vi "WaveformDataTypeTest.vi"() -> ()   [LabVIEW 2017]
uses:
  <userlib>/_OpenG.lib/lvdata/lvdata.llb/Waveform Subtype Enum__ogtk.ctl
panel:
  out "Waveform Subtype Enum":T1 format="%.0x"
  out "StreamTrace":waveform(dbl)(graph)={"t0"=timestamp(1099.9 s since 1904-01-01), "dt"=0.09999999999990905, "Y"=array[30001 elements]} caption="Stream"
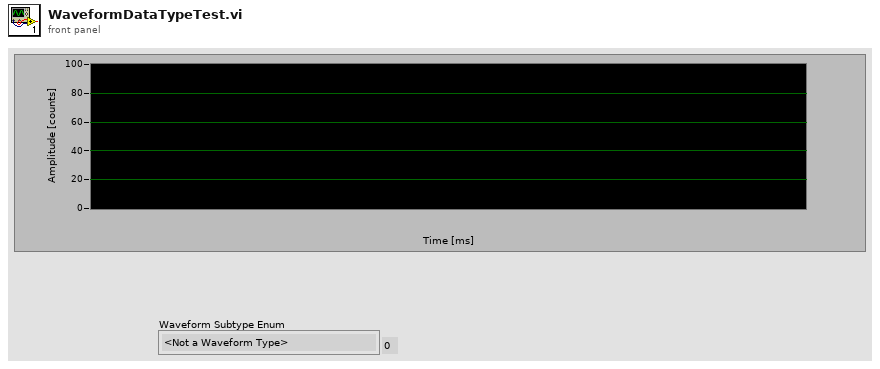
[diagram p1: front panel]
types:
  T1 = typedef "Waveform Subtype Enum__ogtk.ctl" = enum8{"<Not a Waveform Type>", "0x01", "Analog 16-bit signed", "Analog Double-Precision", "0x04", "Analog Single Precision", "Timestamp", "Digital Data", "Digital Waveform", "Dynamic Data", "Analog Extended-Precision", "Analog 8-bit unsigned", "Analog 16-bit unsigned", "Analog 32-bit unsigned", "Analog 8-bit signed", "Analog 32-bit signed", "Analog Complex Single-Precision", "Analog Complex Double-Precision", "Analog Complex Extended Precision", "Analog 64-bit signed", "Analog 64-bit unsigned"}
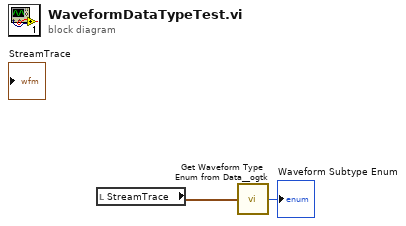
[diagram p0: block diagram]
diagram:
  n1 = local read "StreamTrace"() -> (w2:waveform(dbl))
  n2 = call <userlib>:"Get Waveform Type Enum from Data__ogtk.vi"("Data"=w2) -> ("Waveform Subtype Enum"=→"Waveform Subtype Enum":T1)  [unwired: 4 in]
